vi "QI_AsyncGrab.vi"(7 "path to dll":path, 8 "error in (no error)":errorcluster, 10 "UserEventRef":refnum<user-event>, 11 "Camera Handle":u32) -> (0 "error out":errorcluster, 1 "Frame Address":u32, 2 "Buffer Address":u32, 3 "Camera Handle":u32)   [LabVIEW 2014]
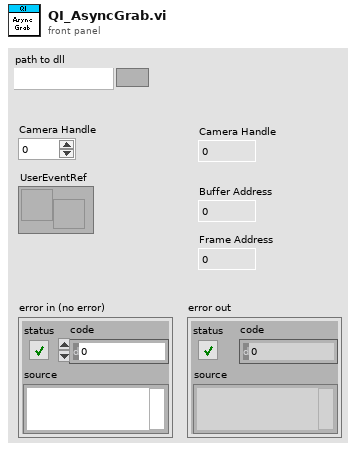
[diagram p1: front panel]
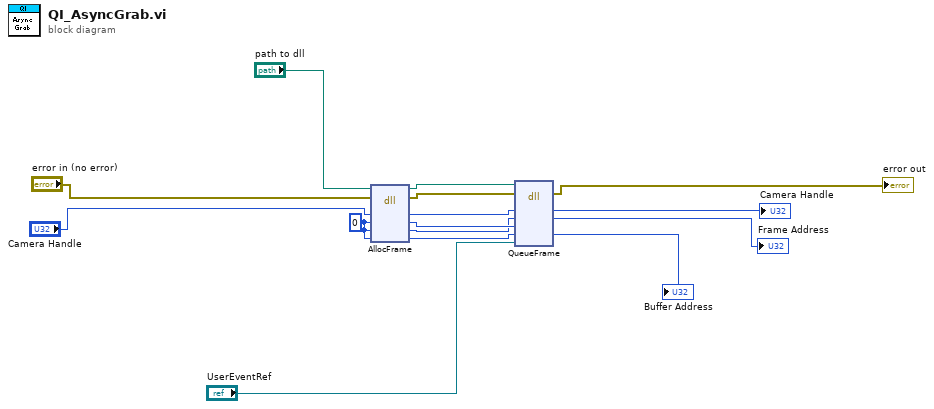
[diagram p0: block diagram]
diagram:
  w15 = u32 0 ("sizeOfBuf")
  n1 = dll-call lib="C:/Users/appli/Documents/Aline/octo-labview/QImaging/Release/QImaging.dll" fn="AllocFrame"(path in="path to dll", error in="error in (no error)", "handle"="Camera Handle", "sizeOfBuf"=w15, "pFrame"=w15, "pBuf"=w15) -> (path out=w1:path, error out=w14:errorcluster, "handle"=w13:u32, "sizeOfBuf"=w12:u32, "pFrame"=w11:u32, "pBuf"=w10:u32)  [unwired: 2 in]
  n2 = dll-call lib="C:/Users/appli/Documents/Aline/octo-labview/QImaging/Release/QImaging.dll" fn="QueueFrame"(path in=w1, error in=w14, "handle"=w13, "pFrame"=w11, "bufferSize"=w12, "pBuf"=w10, "UserEventRef"="UserEventRef") -> (error out=→"error out":errorcluster, "handle"=→"Camera Handle":u32, "pFrame"=→"Frame Address":u32, "pBuf"=→"Buffer Address":u32)  [unwired: 4 in, 1 out]
